vi "Add Widget to Container.vi"(5 "Container":refnum<class "QWidget.lvclass">, 8 "Error In":errorcluster, 9 "Label":string, 10 "Widget":refnum<class "QWidget.lvclass">, 11 "MDI Area Builder in":refnum<class "MDI Area Builder.lvclass">) -> (0 "Error Out":errorcluster, 3 "MDI Area Builder out":refnum<class "MDI Area Builder.lvclass">)   [LabVIEW 2014, in "MDI Area Builder.lvclass"]
doc: "Implements the interface provided by Abstract Widget Builder.\n\n\nCopyright (c) 2019 Sze Howe Koh.\nThis code is licensed under the MIT license."
uses:
  MDI Area Builder.lvclass
  <vilib>/addons/LQ/Qt Widgets/QWidget/QWidget.lvclass
  <vilib>/addons/LQ/Qt Widgets/QMdiArea/QMdiArea.lvclass
  <vilib>/addons/LQ/Qt Widgets/QWidget/setVisible.vi
  <vilib>/addons/LQ/Qt Widgets/QMdiSubWindow/QMdiSubWindow.lvclass
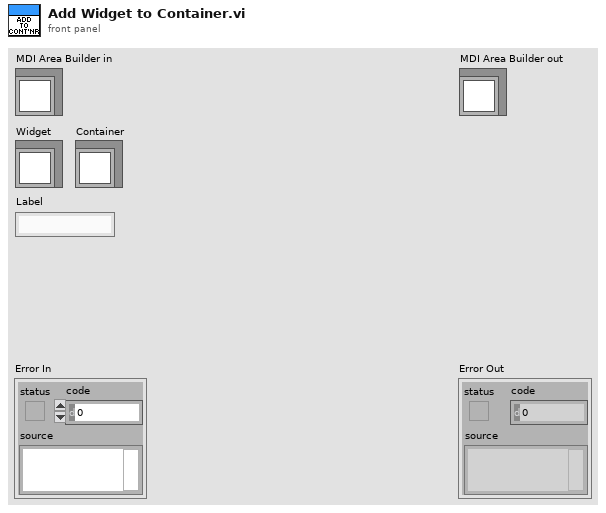
[diagram p1: front panel]
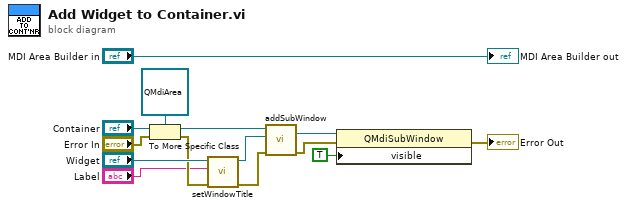
[diagram p0: block diagram]
diagram:
  n1 = To More Specific Class(target class=refnum<class "QMdiArea.lvclass"> refnum ("QMdiArea In"), reference="Container", error in="Error In") -> (specific class reference=w11:refnum<class "QMdiArea.lvclass">, error out=w9:errorcluster)
  n2 = call <vilib>:"setWindowTitle.vi"("Error In"=w9, "windowTitle"="Label", "QWidget In"="Widget") -> ("Error Out"=w6:errorcluster, "QWidget Out"=w7:refnum<class "QWidget.lvclass">)  [unwired: 7 in]
  n3 = call <vilib>:"addSubWindow.vi"("Error In"=w6, "widget"=w7, "QMdiArea In"=w11) -> ("Error Out"=w3:errorcluster, "Value"=w4:refnum<class "QMdiSubWindow.lvclass">)  [unwired: 6 in, 1 out]
  n4 = property class="QMdiSubWindow"(reference=w4, error in=w3, "visible"=TRUE) -> (error out=→"Error Out":errorcluster)  [unwired: 1 out]
  "MDI Area Builder out" <- "MDI Area Builder in"
